vi "Serialize.vi"(8 "error in (no error)":errorcluster, 11 "ADAS PE Template Controller in":refnum<class "PE Controller.lvclass">) -> (0 "error out":errorcluster, 2 "Serialized PE Specification":string, 3 "ADAS PE Template Controller out":refnum<class "PE Controller.lvclass">)   [LabVIEW 2020, in "ADAS PE Template.lvlib" / "PE Controller.lvclass"]
doc: "<b>Serialize</b>\nProvides the seralized configuration data stored in the plugin controller's class data."
uses:
  PE Controller.lvclass
  PE Controller.lvclass/PE Controller.ctl
  PE/Get Configuration Version.vi
  <vilib>/ADAS Record/Utilities/Config/Data Converter/Data Container and Version to JSON.vi
  PE/ADAS PE Template.lvclass
panel:
  # "#via_ignore"
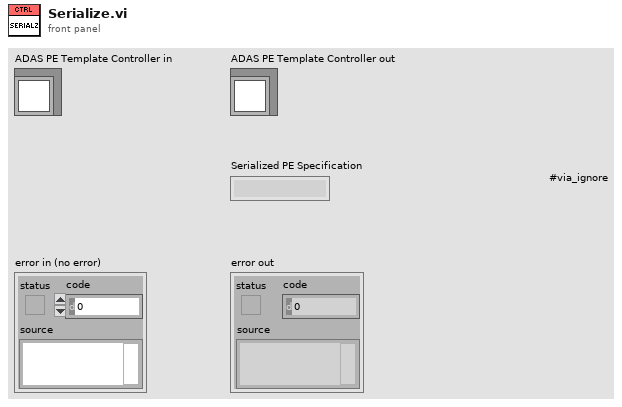
[diagram p1: front panel]
types:
  T1 = typedef "ADAS PE Template.lvlib/ADAS PE Template.lvclass/Configuration.ctl" = cluster{"Parameter1":string}
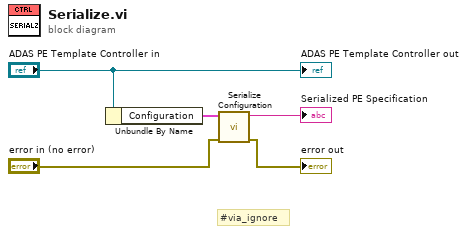
[diagram p0: block diagram]
diagram:
  # "#via_ignore"
  n1 = Unbundle By Name("ADAS PE Template Controller in") -> ("Configuration"=w4:T1)
  n2 = call "Serialize Configuration.vi"("error in (no error)"="error in (no error)", "Configuration"=w4) -> ("error out"=→"error out":errorcluster, "Serialized Configuration"=→"Serialized PE Specification":string)  [unwired: 8 in]
  "ADAS PE Template Controller out" <- "ADAS PE Template Controller in"
